vi "SloweTimeAverage.vi"(8 "index":i32, 10 "Filtered Out":csg[][][](array[numeric]), 11 "Average":i32=3) -> (2 "Slow Average":csg[][](array[numeric]))   [LabVIEW 2022 SP3]
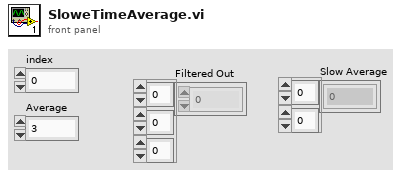
[diagram p1: front panel]
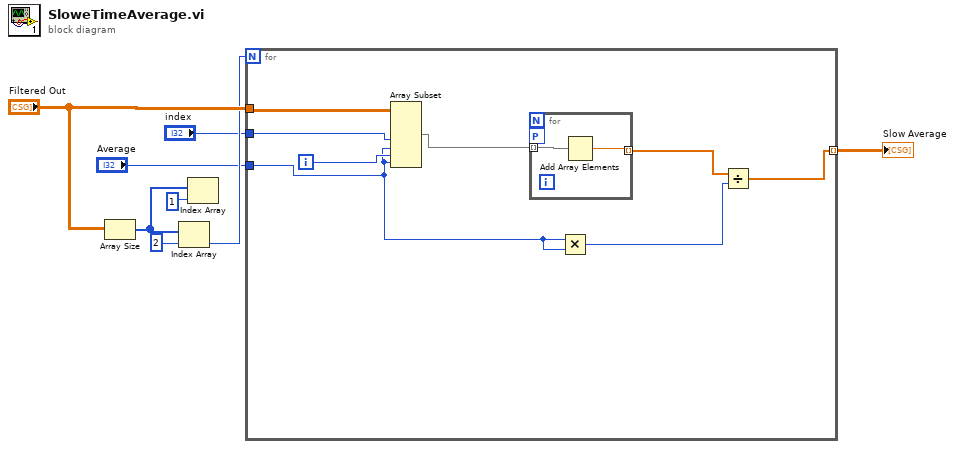
[diagram p0: block diagram]
diagram:
  n1 = Array Size(array="Filtered Out") -> (size(s)=w7:i32[])
  n2 = Index Array(array=w7, index=2) -> (element=w4:i32)
  n3 = Index Array(array=w7, index=1) -> ()  [unwired: 1 out]
  n4 = for {
    N: w4 -> [_]
    tunnel: "Filtered Out" -> [w16]
    tunnel: "index" -> [w13]
    tunnel: [w10] -> w2 mode=indexing
    tunnel: "Average" -> [w9]
    i -> [w14]
    n5 = Array Subset(array=w16, index (dim 1)=w13, length (dim 1)=w9, index (dim 2)=w14, length (dim 2)=w9) -> (w15:csg[][][])  [unwired: 2 in]
    n6 = for {
      tunnel: w15 -> [w18] mode=indexing
      tunnel: [w17] -> w12 mode=indexing
      workers-P: _ -> [_]
      n7 = Add Array Elements(numeric array=w18) -> (sum=w17:csg)
    }
    n8 = Multiply(x=w9, y=w9) -> (x*y=w11:i32)
    n9 = Divide(x=w12, y=w11) -> (x/y=w10:csg[])
  }
  "Slow Average" <- w2
